vi "MP - add Pos and MIP to encoder status.vi"(9 "Axis Status":T1 {"IO Levels"."Outputs: 7-0" format="%.0b"; "IO Levels"."Outputs: 15-8" format="%.0b"; "IO Levels"."Inputs: 7-0" format="%.0b"; "IO Levels"."Inputs: 15-8" format="%.0b"}, 11 "scan data info":T3={"Message Header"=0, "Error Message"=0, "Test No."=0, "Channel No."=0, "Sweep No."=0, "Gate No."=0, "DOF"=enum."", "retain data"=enum."Ascan", "scan data"=[], "scan length"=0, "scan index"=0, "peak data"={"timebase"=[], "data"=[]}, "#peaks"=0, "PRF"=0.0, "IP"={"Axis No."=0, "Location"=0, "MIP location"=0, "MIP?"=FALSE}, "echo range"=0, "ETG"=FALSE, "CAL 0 complete"=FALSE, "Axis Positions"={"Axis 1"=0, "Axis 2"=0, "Axis 3"=0, "Axis 4"=0, "Status"=0}} {"Error Message" format="%04x"; "Message Header" format="%04x"; "IP"."MIP location" format="%#.0f"; "IP"."Location" format="%#.0f"; "PRF" format="%.0fHz"}) -> (3 "scan data info":T3={"Message Header"=0, "Error Message"=0, "Test No."=0, "Channel No."=0, "Sweep No."=0, "Gate No."=0, "DOF"=enum."", "retain data"=enum."Ascan", "scan data"=[], "scan length"=0, "scan index"=0, "peak data"={"timebase"=[], "data"=[]}, "#peaks"=0, "PRF"=0.0, "IP"={"Axis No."=0, "Location"=0, "MIP location"=0, "MIP?"=FALSE}, "echo range"=0, "ETG"=FALSE, "CAL 0 complete"=FALSE, "Axis Positions"={"Axis 1"=0, "Axis 2"=0, "Axis 3"=0, "Axis 4"=0, "Status"=0}} {"Error Message" format="%04x"; "Message Header" format="%04x"; "IP"."MIP location" format="%#.0f"; "IP"."Location" format="%#.0f"; "PRF" format="%.0fHz"})   [LabVIEW 2026, in "MicroPulse_Driver.lvlib"]
uses:
  MicroPulse_Driver.lvlib
  Public/Data/Datatypes/MP - scan data info.ctl
  Public/Data/Datatypes/MP - data output format.ctl
  Public/Data/Datatypes/MP - retain scan.ctl
  Public/Data/Datatypes/MP - axis positions (LLC).ctl
  Public/Data/Datatypes/MP - axis status.ctl
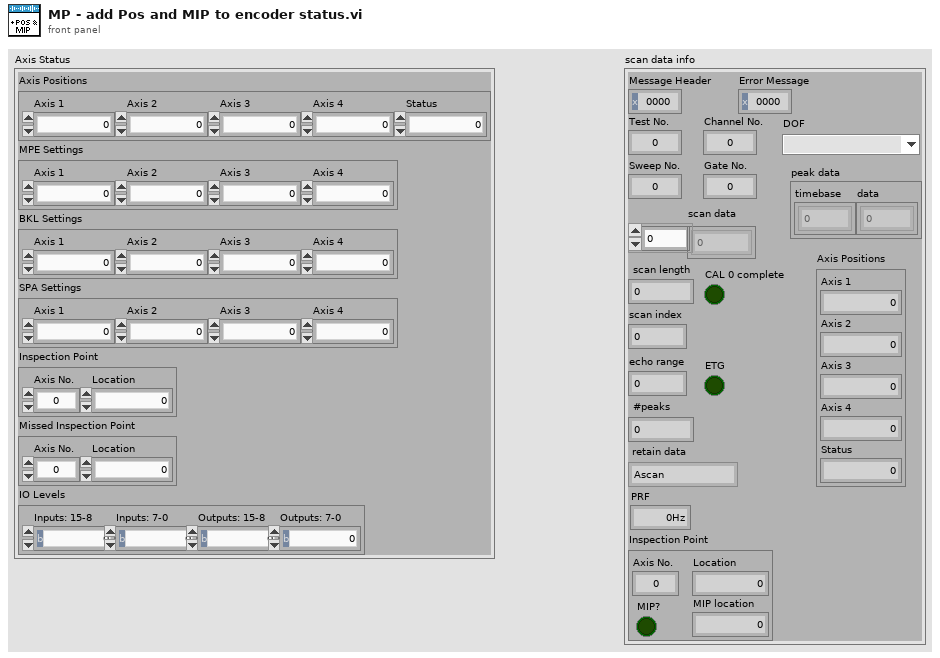
[diagram p1: front panel]
types:
  T1 = typedef "MicroPulse_Driver.lvlib/MP - axis status.ctl" = cluster{"Axis Positions":T2, "MPE Settings":cluster{"Axis 1":u32, "Axis 2":u32, "Axis 3":u32, "Axis 4":u32}, "BKL Settings":cluster{"Axis 1":u32, "Axis 2":u32, "Axis 3":u32, "Axis 4":u32}, "SPA Settings":cluster{"Axis 1":u32, "Axis 2":u32, "Axis 3":u32, "Axis 4":u32}, "IP":cluster{"Axis No.":u8, "Location":u32}, "MIP":cluster{"Axis No.":u8, "Location":u32}, "IO Levels":cluster{"Inputs: 15-8":u8, "Inputs: 7-0":u8, "Outputs: 15-8":u8, "Outputs: 7-0":u8}}
  T2 = typedef "MicroPulse_Driver.lvlib/MP - axis positions (LLC).ctl" = cluster{"Axis 1":u32, "Axis 2":u32, "Axis 3":u32, "Axis 4":u32, "Status":u8}
  T3 = typedef "MicroPulse_Driver.lvlib/MP - scan data info.ctl" = cluster{"Message Header":u16, "Error Message":u16, "Test No.":u32, "Channel No.":u8, "Sweep No.":u32, "Gate No.":u32, "DOF":T4, "retain data":T5, "scan data":u16[], "scan length":i32, "scan index":i32, "peak data":cluster{"timebase":u16[], "data":u16[]}, "#peaks":i32, "PRF":dbl, "IP":cluster{"Axis No.":u8, "Location":u32, "MIP location":u32, "MIP?":bool}, "echo range":u16, "ETG":bool, "CAL 0 complete":bool, "Axis Positions":T2}
  T4 = typedef "MicroPulse_Driver.lvlib/MP - data output format.ctl" = enum16{"", "8-bit Mode", "10-bit Mode", "12-bit Mode", "16-bit Mode", "8-bit Log Mode", "12-bit Packed Mode"}
  T5 = typedef "MicroPulse_Driver.lvlib/MP - retain scan.ctl" = enum16{"None", "Ascan", "Peaks"}
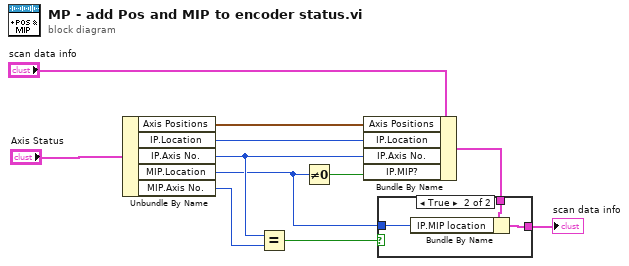
[diagram p0: block diagram]
diagram:
  n1 = Unbundle By Name("Axis Status") -> ("Axis Positions"=w1:T2, "IP.Location"=w10:u32, "IP.Axis No."=w9:u8, "MIP.Location"=w3:u32, "MIP.Axis No."=w2:u8)
  n2 = Equal?(x=w9, y=w2) -> (x = y?=w5:bool)
  n3 = Not Equal To 0?(x=w3) -> (x != 0?=w4:bool)
  n4 = Bundle By Name(cluster="scan data info", "Axis Positions"=w1, "IP.Location"=w10, "IP.Axis No."=w9, "IP.MIP?"=w4) -> (w7:T3)
  n5 = case shown="True" w5 {
    tunnel: w7 -> [w12 w15]
    tunnel: [w12 w14] -> w6
    tunnel: w3 -> [_ w13]
    frame False {
    }
    frame True {
      n6 = Bundle By Name(cluster=w15, "IP.MIP location"=w13) -> (w14:T3)
    }
  }
  "scan data info" <- w6
